vi "Extrae_Measure.vi"(10 "String":string="                Measure 30 seconds or 10 points every 1 seconds, 10 averages") -> (1 "Array":string[](array[string]))   [LabVIEW 2017]
panel:
  # "Measure for 0.001 seconds every 0.100 seconds, 1 averages"
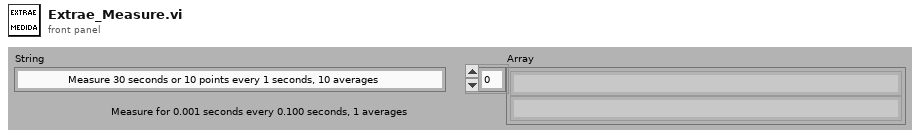
[diagram p1: front panel]
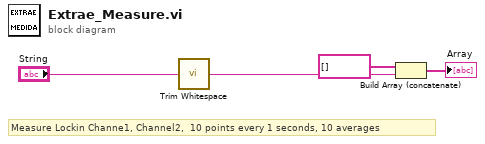
[diagram p0: block diagram]
diagram:
  # "Measure Lockin Channe1, Channel2,  10 points every 1 seconds, 10 averages"
  n1 = call <vilib>:"Trim Whitespace.vi"("string"="String") -> ("trimmed string"=w1:string)  [unwired: 1 in]
  n2 = Build Array (concatenate)(string[] [] ("Array I"), w1) -> (→"Array":string[])
